vi "Control Label.vi"(8 "error in (no error)":errorcluster, 9 "operation":enum16{"Get", "Set"}(ring), 11 "label":string) -> (0 "error out":errorcluster, 3 "label out":string)   [LabVIEW 2018, in "NISAST VI Scripting.lvlib" / "VI.lvlib" / "Front Panel.lvlib"]
uses:
  Front Panel.lvlib
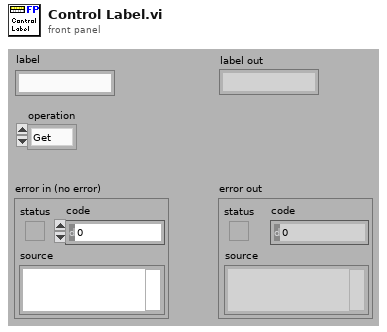
[diagram p1: front panel]
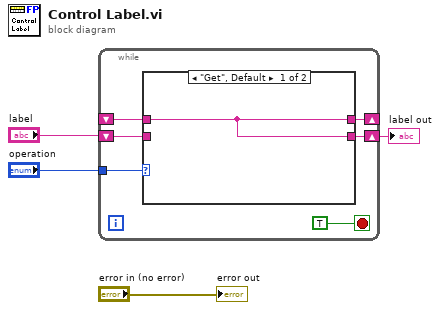
[diagram p0: block diagram]
diagram:
  n1 = while {
    shift-right: [w10] -> _
    shift-left: _ -> [w9]
    shift-right: [w7] -> w3
    shift-left: "label" -> [w8]
    tunnel: "operation" -> [w5]
    stop <- TRUE stop-if-true
    n2 = case shown="\"Get\", Default" w5 {
      tunnel: [w11 w12] -> w10
      tunnel: w9 -> [w11 _]
      tunnel: w8 -> [_ w12]
      tunnel: [w11 w12] -> w7
      frame "Get", Default {
      }
      frame "Set" {
      }
    }
  }
  "label out" <- w3
  "error out" <- "error in (no error)"
